vi "编制工艺.vi"(8 "error in (no error)":errorcluster caption="错误输入（无错误）", 11 "零件加工（抽象） 输入":refnum<class "零件加工（抽象）.lvclass"> caption="DNL_LabVIEW Object in") -> (0 "error out":errorcluster caption="错误输出", 2 "编制工艺":string, 3 "零件加工（抽象） 输出":refnum<class "零件加工（抽象）.lvclass"> caption="DNL_LabVIEW Object out")   [LabVIEW 2013, in "零件加工（抽象）.lvclass"]
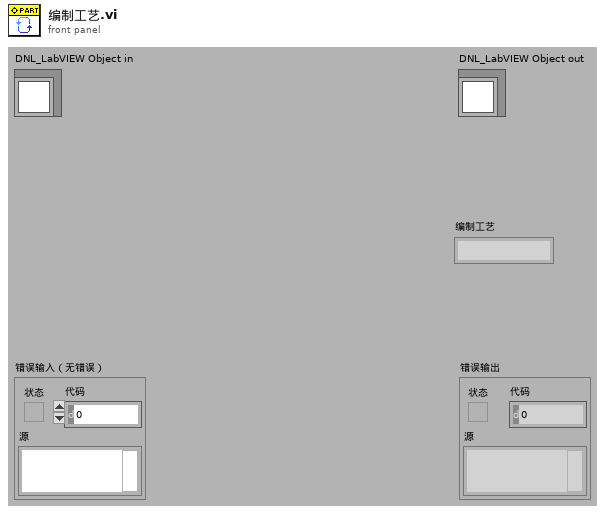
[diagram p1: front panel]
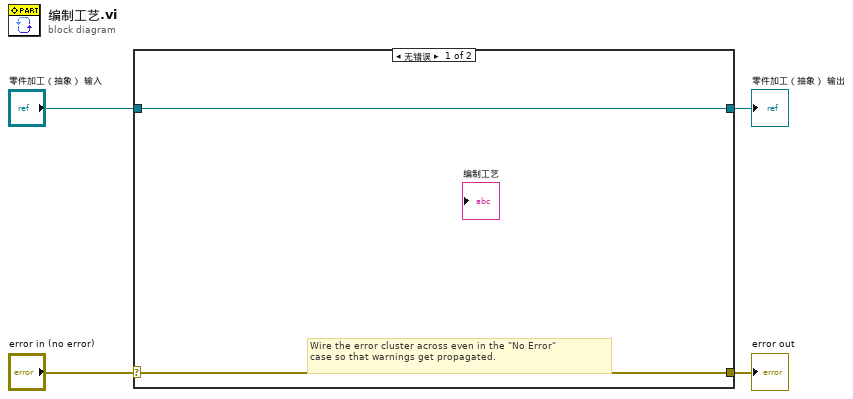
[diagram p0: block diagram]
diagram:
  n1 = case shown="无错误" "error in (no error)" {
    selector: "error in (no error)" -> [w5 w8]
    tunnel: [w5 w8] -> w3
    tunnel: [w6 w7] -> w1
    tunnel: "零件加工（抽象） 输入" -> [w6 w7]
    frame No Error {
      # "Wire the error cluster across even in the \"No Error\"\ncase so that warnings get propagated."
    }
    frame Error {
    }
  }
  "error out" <- w3
  "零件加工（抽象） 输出" <- w1
